vi "solar_tcp Debug Set.vi"(7 "Action":T4, 8 "error in (no error)":errorcluster, 9 "Update? (T)":bool=TRUE, 10 "Message Sent/Read":string, 11 "TCP Data in":T1={"Connected"=FALSE, "Config"={"TCPServer"=enum."SERVER", "ServerPort"=0, "IPAddress"="", "ClientPort"=0, "HdrSizeBytes"=4, "HdrLenSubtractBytes"=0, "HdrLenOffsetBits"=0, "HdrLenSizeBits"=32}, "Clients"=[], "ConnectionID"=refnum, "Debug"=[]} {"Debug"."Time" format="%<%Y-%m-%d\n%H:%M:%S%3u>T"}) -> (0 "error out":errorcluster, 3 "TCP Data out":T1={"Connected"=FALSE, "Config"={"TCPServer"=enum."SERVER", "ServerPort"=0, "IPAddress"="", "ClientPort"=0, "HdrSizeBytes"=4, "HdrLenSubtractBytes"=0, "HdrLenOffsetBits"=0, "HdrLenSizeBits"=32}, "Clients"=[], "ConnectionID"=refnum, "Debug"=[]} {"Debug"."Time" format="%<%Y-%m-%d\n%H:%M:%S%3u>T"})   [LabVIEW 2018]
doc: "This sets the TCP debug log. The debug log maintains the last 100 elements."
uses:
  solar_tcp_ctl Action.ctl
  solar_tcp_ctl Debug.ctl
  solar_tcp_ctl Config.ctl
  solar_tcp_ctl Data.ctl
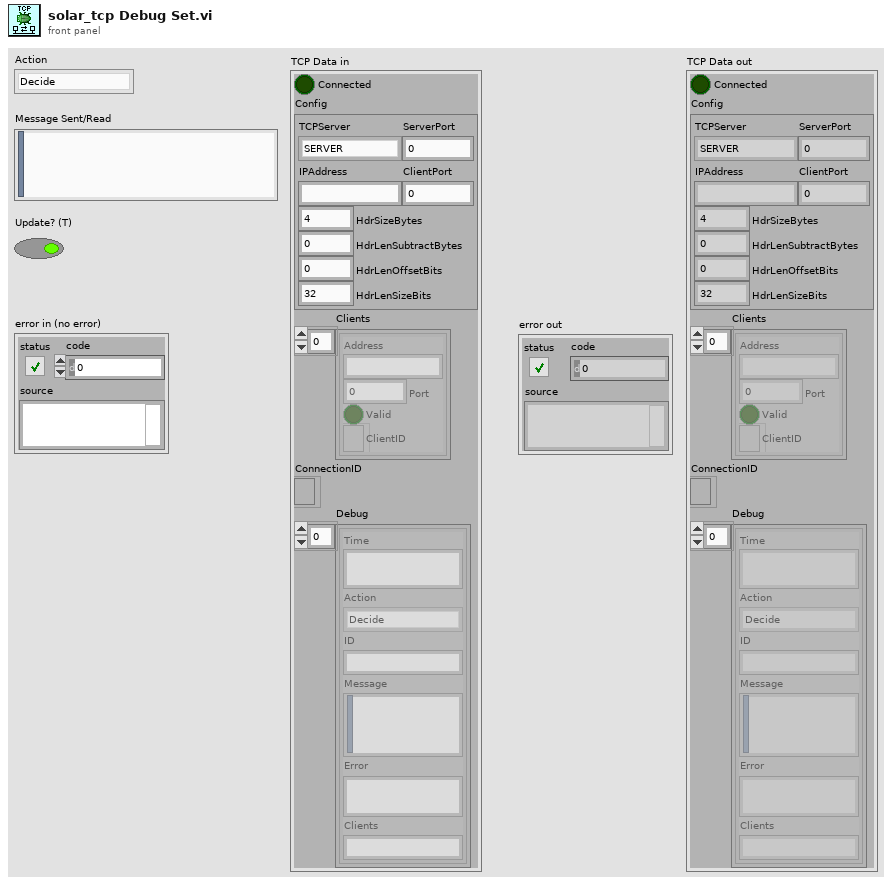
[diagram p1: front panel]
types:
  T1 = typedef "solar_tcp_ctl Data.ctl" = cluster{"Connected":bool, "Config":T2, "Clients":cluster{"Address":string, "Port":u16, "Valid":bool, "ClientID":refnum<k5>}[], "ConnectionID":refnum<k5>, "Debug":T3[]}
  T2 = typedef "solar_tcp_ctl Config.ctl" = cluster{"TCPServer":enum8{"SERVER", "CLIENT"}, "ServerPort":u16, "IPAddress":string, "ClientPort":u16, "HdrSizeBytes":i32, "HdrLenSubtractBytes":i32, "HdrLenOffsetBits":i32, "HdrLenSizeBits":i32}
  T3 = typedef "solar_tcp_ctl Debug.ctl" = cluster{"Time":timestamp, "Action":T4, "ID":string, "Message":string, "Error":string, "Clients":string}
  T4 = typedef "solar_tcp_ctl Action.ctl" = enum16{"Decide", "CreateListener", "Open", "Read", "Write", "Close", "Shutdown", "Done", "ChangePort"}
  T5 = cluster{"Address":string, "Port":u16, "Valid":bool, "ClientID":refnum<k5>}[]
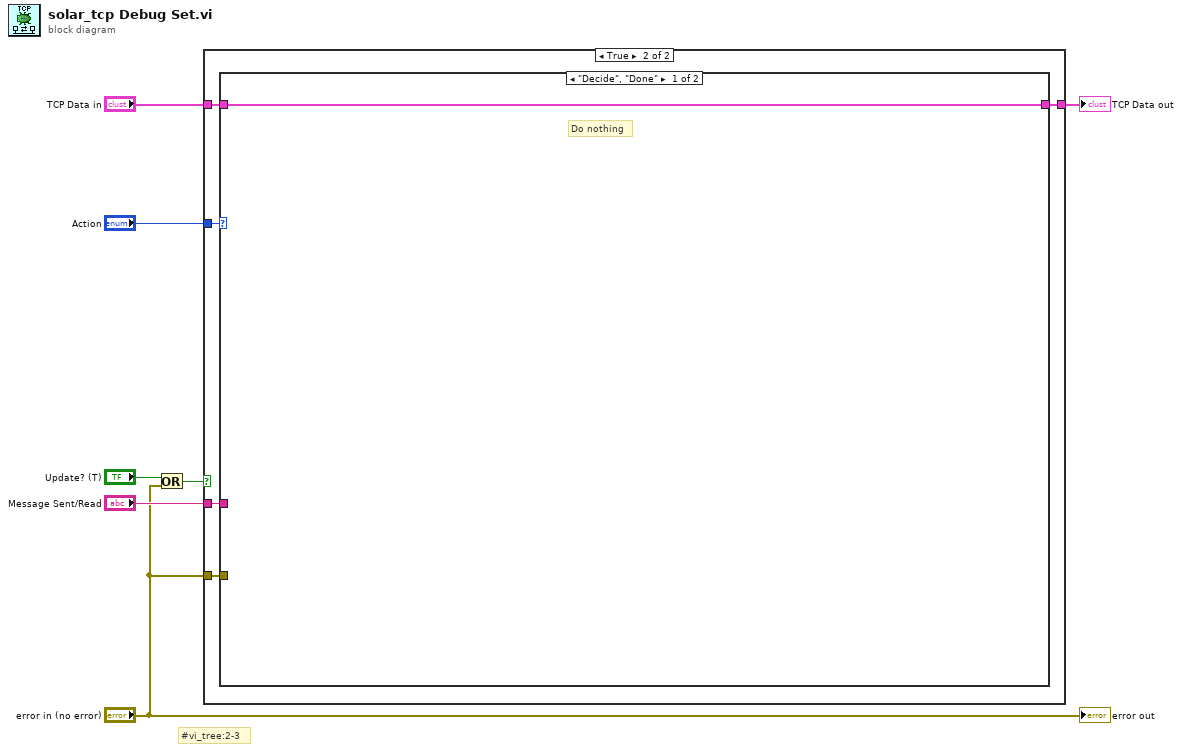
[diagram p0: block diagram]
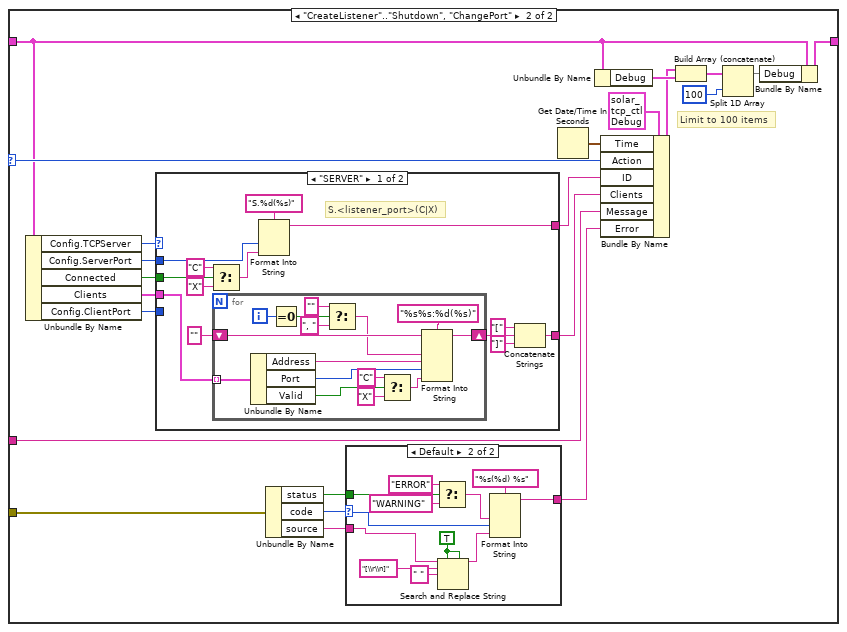
[diagram p3: hidden frame]
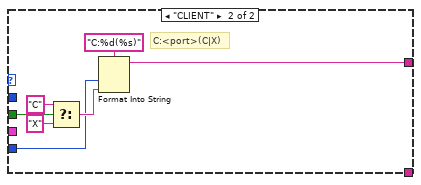
[diagram p4: hidden frame]
diagram:
  # "#vi_tree:2-3"
  n1 = Or(x="Update? (T)", y="error in (no error)") -> (x .or. y?=w2:bool)
  n2 = case shown="True" w2 {
    tunnel: "Message Sent/Read" -> [_ w13]
    tunnel: "error in (no error)" -> [_ w12]
    tunnel: "TCP Data in" -> [w8 w11]
    tunnel: "Action" -> [_ w10]
    tunnel: [w8 w9] -> w4
    frame False {
    }
    frame True {
      n3 = case shown="\"Decide\", \"Done\"" w10 {
        selector: w10 -> [_ w36]
        tunnel: w11 -> [w14 w33]
        tunnel: w13 -> [_ w34]
        tunnel: w12 -> [_ w37]
        tunnel: [w14 w35] -> w9
        frame "Decide", "Done" {
          # "Do nothing"
        }
        frame "CreateListener".."Shutdown", "ChangePort" {
          # "Limit to 100 items"
          n4 = Unbundle By Name(w33) -> ("Config.TCPServer"=w31:enum8{"SERVER", "CLIENT"}, "Config.ServerPort"=w30:u16, "Connected"=w29:bool, "Clients"=w32:T5, "Config.ClientPort"=w28:u16)
          n5 = case shown="\"SERVER\"" w31 {
            tunnel: [w42 w71] -> w23
            tunnel: w32 -> [w49 _]
            tunnel: w30 -> [w47 _]
            tunnel: w29 -> [w44 w68]
            tunnel: w28 -> [_ w66]
            tunnel: [w40 _] -> w20
            frame "SERVER" {
              # "S.<listener_port>(C|X)"
              n6 = Select(t="C", s=w44, f="X") -> (s? t:f=w43:string)
              n7 = for {
                tunnel: w49 -> [w65] mode=indexing
                shift-right: [w61] -> w41
                shift-left: "" -> [w60]
                i -> [w55]
                n8 = Unbundle By Name(w65) -> ("Address"=w63:string, "Port"=w62:u16, "Valid"=w57:bool)
                n9 = Equal To 0?(x=w55) -> (x = 0?=w54:bool)
                n10 = Select(t="", s=w54, f=", ") -> (s? t:f=w51:string)
                n11 = Select(t="C", s=w57, f="X") -> (s? t:f=w56:string)
                n12 = Format Into String(format string="%s%s:%d(%s)", initial string=w60, w51, w63, w62, w56) -> (resulting string=w61:string)  [unwired: 1 in, 1 out]
              }
              n13 = Format Into String(format string="S.%d(%s)", w47, w43) -> (resulting string=w42:string)  [unwired: 2 in, 1 out]
              n14 = Concatenate Strings("[" ("string"), w41, "]" ("string")) -> (w40:string)
            }
            frame "CLIENT" {
              # "C:<port>(C|X)"
              n15 = Select(t="C", s=w68, f="X") -> (s? t:f=w67:string)
              n16 = Format Into String(format string="C:%d(%s)", w66, w67) -> (resulting string=w71:string)  [unwired: 2 in, 1 out]
            }
          }
          n17 = Unbundle By Name(w37) -> ("status"=w26:bool, "code"=w27:i32, "source"=w25:string)
          n18 = case shown="Default" w27 {
            selector: w27 -> [_ w80]
            tunnel: w26 -> [_ w84]
            tunnel: w25 -> [_ w77]
            tunnel: [_ w78] -> w22
            frame 0 {
            }
            frame Default {
              w74 = TRUE ("replace all? (F)")
              n19 = Select(t="ERROR", s=w84, f="WARNING") -> (s? t:f=w81:string)
              n20 = Search and Replace String(replace all?=w74, multiline?=w74, input string=w77, search string="[\\r\\n]", replace string=" " ("replace string (\"\")")) -> (result string=w76:string)  [unwired: 3 in, 3 out]
              n21 = Format Into String(format string="%s(%d) %s", w81, w80, w76) -> (resulting string=w78:string)  [unwired: 2 in, 1 out]
            }
          }
          n22 = Get Date/Time In Seconds() -> (seconds since 1Jan1904=w21:timestamp)
          n23 = Unbundle By Name(w33) -> ("Debug"=w19:T3[])
          n24 = Bundle By Name(cluster=T3 {"Time"=timestamp(0 s since 1904-01-01), "Action"=enum."Decide", "ID"="", "Message"="", "Error"="", "Clients"=""} ("Debug"), "Time"=w21, "Action"=w36, "ID"=w23, "Clients"=w20, "Message"=w34, "Error"=w22) -> (w18:T3)
          n25 = Build Array (concatenate)(w18, w19) -> (w17:T3[])
          n26 = Split 1D Array(array=w17, index=100) -> (first subarray=w16:T3[])  [unwired: 1 out]
          n27 = Bundle By Name(cluster=w33, "Debug"=w16) -> (w35:T1)
        }
      }
    }
  }
  "TCP Data out" <- w4
  "error out" <- "error in (no error)"
